vi "Frame Update GoTo.vi"(8 "error in (no error)":errorcluster, 11 "LF2R IDE in":refnum<class "LF2R IDE.lvclass">) -> (0 "error out":errorcluster, 3 "LF2R IDE out":refnum<class "LF2R IDE.lvclass">)   [LabVIEW 2018, in "LF2R IDE.lvlib" / "LF2R IDE.lvclass"]
uses:
  LF2R IDE.lvclass
  LF2R IDE.lvclass/LF2R IDE.ctl
  ScintillaNET/ScintillaNET.lvclass
  Frame Analizer/Data Parser.lvclass
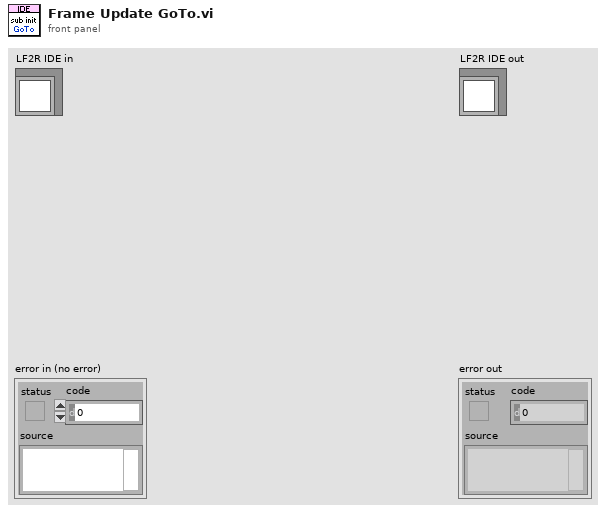
[diagram p1: front panel]
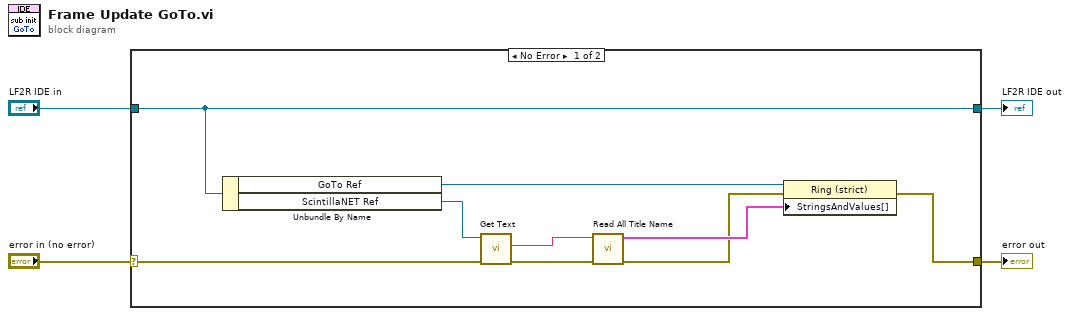
[diagram p0: block diagram]
diagram:
  n1 = case shown="No Error" "error in (no error)" {
    selector: "error in (no error)" -> [w10 w15]
    tunnel: [w5 w15] -> w3
    tunnel: [w12 w14] -> w1
    tunnel: "LF2R IDE in" -> [w12 w14]
    frame No Error {
      n2 = Unbundle By Name(w12) -> ("GoTo Ref"=w13:refnum<vi>, "ScintillaNET Ref"=w11:refnum<class "ScintillaNET.lvclass">)
      n3 = call "Get Text.vi"("error in (no error)"=w10, "ScintillaNET in"=w11) -> ("error out"=w8:errorcluster, "Text"=w9:string)  [unwired: 7 in, 1 out]
      n4 = call "Read All Title Name.vi"("error in (no error)"=w8, "File String"=w9) -> ("error out"=w6:errorcluster, "Title Name and Frame Num"=w7:cluster{"Name":string, "Num":i32}[])  [unwired: 8 in]
      n5 = property class="Ring (strict)"(reference=w13, error in=w6, "StringsAndValues[]"=w7) -> (error out=w5:errorcluster)  [unwired: 1 out]
    }
    frame Error {
    }
  }
  "error out" <- w3
  "LF2R IDE out" <- w1
